vi "Hold.vi"(8 "error in (no error)":errorcluster, 10 "Hold (T: Enable)":bool=TRUE, 11 "VISA resource name":refnum<visa-resource-name>) -> (0 "error out":errorcluster, 3 "VISA resource name out":refnum<visa-resource-name>)   [LabVIEW 2021, in "Yokogawa WT1800 Series.lvlib"]
doc: "The hold operation stops data measurement and display operations for each data update interval and holds the display of all measurement function data. The D/A output values, the values in the data lists printed by the builtin printer, and the communication values all reflect the held values."
uses:
  <instrlib>/Yokogawa WT1800 Series/Yokogawa WT1800 Series.lvlib
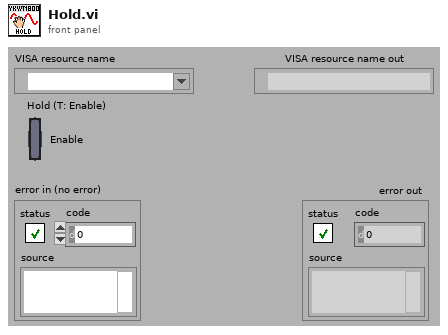
[diagram p1: front panel]
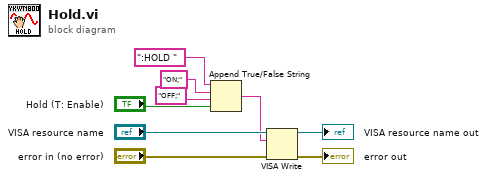
[diagram p0: block diagram]
diagram:
  n1 = Append True/False String ("True/False 文字列を追加")(1:"Hold (T: Enable)", 2:"OFF;", 3:"ON;", 4:":HOLD ") -> (0:w2:string)
  n2 = VISA Write ("VISA書き込み")(VISA resource name="VISA resource name", write buffer=w2, error in (no error)="error in (no error)") -> (VISA resource name out=→"VISA resource name out":refnum<visa-resource-name>, error out=→"error out":errorcluster)  [unwired: 1 out]
